vi "Module Setup.vi"(6 "Invert":bool, 8 "Vel ID 2":u8, 9 "Vel ID":u8, 10 "Rot ID":u8, 11 "Mod Des":string) -> ()   [LabVIEW 2020]
doc: "vi to set up the swerve modules using spark max , rev through bore encoder and internal encoder"
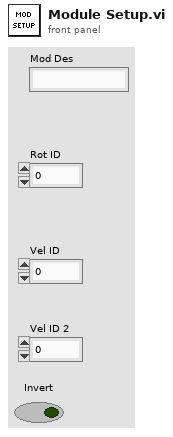
[diagram p1: front panel]
types:
  T1 = typedef "WPI_MotorControlDeviceRef.ctl" = cluster{"DeviceStatus":errorcluster, "Type":T2, "PWM":cluster{"PWM Channel":T3, "DeadBand":T4}, "CAN":cluster{"Device Number":u8, "SetOutput VI Ref":variant, "GetOutput VI Ref":variant, "Enable VI Ref":variant, "Disable VI Ref":variant, "Data":variant}, "Invert":bool, "DIO PWM":cluster{"PWM \"Enable\" Channel":T3, "DIOChannel":T5, "PWM Rate":dbl}}
  T2 = typedef "WPI_MotorControlType.ctl" = enum16{"PWM", "CAN", "DIO PWM"}
  T3 = typedef "FPGA_DIOPWMChannel.ctl" = enum8{"PWM 0", "PWM 1", "PWM 2", "PWM 3", "PWM 4", "PWM 5", "PWM 6", "PWM 7", "PWM 8", "PWM 9", "PWM MXP 0", "PWM MXP 1", "PWM MXP 2", "PWM MXP 3", "PWM MXP 4", "PWM MXP 5", "PWM MXP 6", "PWM MXP 7", "PWM MXP 8", "PWM MXP 9", "Invalid"}
  T4 = typedef "WPI_PWMDeadband.ctl" = cluster{"Name":string, "maxPositivePwm":i32, "minPositivePwm":i32, "centerPwm":i32, "maxNegativePwm":i32, "minNegativePwm":i32, "angularRange":u16}
  T5 = typedef "FPGA_DIOChannel.ctl" = enum8{"DIO 0", "DIO 1", "DIO 2", "DIO 3", "DIO 4", "DIO 5", "DIO 6", "DIO 7", "DIO 8", "DIO 9", "DIO MXP 0", "DIO MXP 1", "DIO MXP 2", "DIO MXP 3", "DIO MXP 4", "DIO MXP 5", "DIO MXP 6", "DIO MXP 7", "DIO MXP 8", "DIO MXP 9", "DIO MXP 10", "DIO MXP 11", "DIO MXP 12", "DIO MXP 13", "DIO MXP 14", "DIO MXP 15", "SPI Port CS1", "SPI Port CS2", "SPI Port CS3", "SPI Port MISO", "SPI Port MOSI", "Invalid"}
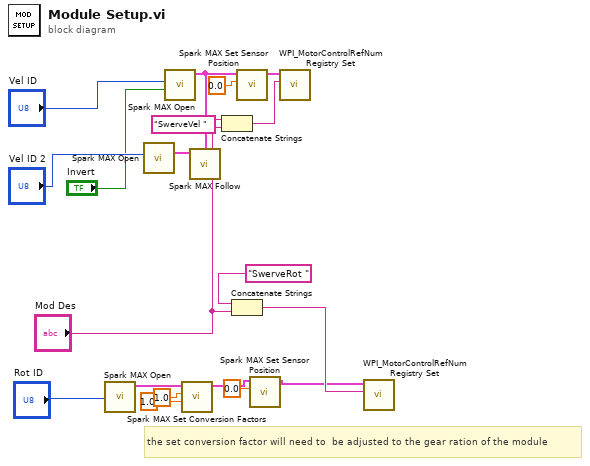
[diagram p0: block diagram]
diagram:
  # "the set conversion factor will need to  be adjusted to the gear ration of the module"
  n1 = call <vilib>:"Spark MAX Open.vi"("Device Number"="Rot ID") -> ("MotorControlDeviceRef"=w10:T1)  [unwired: 9 in, 1 out]
  n2 = call <vilib>:"Spark MAX Open.vi"("Device Number"="Vel ID 2") -> ("MotorControlDeviceRef"=w4:T1)  [unwired: 9 in, 1 out]
  n3 = call <vilib>:"Spark MAX Open.vi"("Invert"="Invert", "Device Number"="Vel ID") -> ("MotorControlDeviceRef"=w3:T1)  [unwired: 8 in, 1 out]
  n4 = call <vilib>:"Spark MAX Set Conversion Factors.vi"("Velocity Factor (1)"=1.0, "Position Factor (1)"=1.0 ("Position Conversion Factor (1)"), "MotorControlDeviceRef in"=w10) -> ("MotorControlDeviceRef out"=w7:T1)  [unwired: 7 in, 1 out]
  n5 = call <vilib>:"Spark MAX Follow.vi"("Master Controller"=w3, "MotorControlDeviceRef"=w4) -> ()  [unwired: 8 in, 2 out]
  n6 = Concatenate Strings("SwerveVel " ("refnum name"), "Mod Des") -> (w18:string)
  n7 = Concatenate Strings("SwerveRot " ("refnum name"), "Mod Des") -> (w19:string)
  n8 = call <vilib>:"Spark MAX Set Sensor Position.vi"("Position"=0.0, "MotorControlDeviceRef"=w3) -> ("MotorControlDeviceRef"=w14:T1)  [unwired: 8 in, 1 out]
  n9 = call <vilib>:"Spark MAX Set Sensor Position.vi"("Position"=0.0, "MotorControlDeviceRef"=w7) -> ("MotorControlDeviceRef"=w8:T1)  [unwired: 8 in, 1 out]
  n10 = call <vilib>:"WPI_MotorControlRefNum Registry Set.vi"("refnum name"=w18, "MotorControlDevRef"=w14) -> ()  [unwired: 8 in, 2 out]
  n11 = call <vilib>:"WPI_MotorControlRefNum Registry Set.vi"("refnum name"=w19, "MotorControlDevRef"=w8) -> ()  [unwired: 8 in, 2 out]
